vi "Process.vi"(8 "error in":errorcluster, 11 "SMO.A":refnum<class "SMO.D.lvclass">) -> (0 "error out":errorcluster, 3 "SMO.A out":refnum<class "SMO.D.lvclass">)   [LabVIEW 2013, in "SMO.D.lvclass"]
doc: "---------------------------------------------------------------\nJKI State Machine Objects™\nhttp://jki.net/state-machine-objects/\nCopyright (C) 2005-2015, JKI <info@jki.net>\nALL RIGHTS RESERVED"
uses:
  SMO.D.lvclass
  src/SMO/Typedefs/Parent Call--Enum.ctl
  src/SMO/SMO.lvclass
panel:
  # "For instructions on how to use the JKI State Machine Objects, examples and video tutorials, visit:\nhttp://jki.net/state-machine-objects/\n\nJKI State Machine Objects™\nhttp://jki.net/state-machine-objects/\nCopyright (C) 2005-2015, JKI <info@jki.net>\nALL RIGHTS RESERVED"
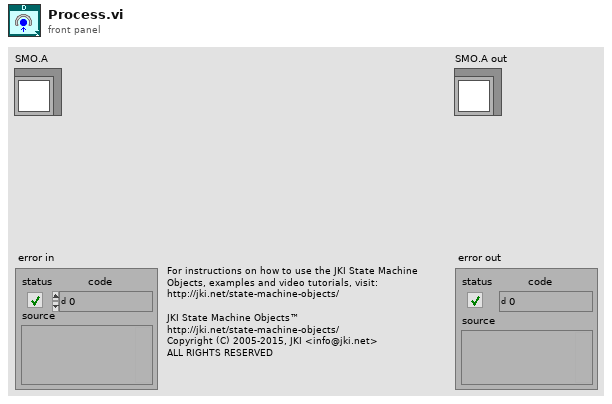
[diagram p1: front panel]
types:
  T1 = typedef "SMO.lvclass/Parent Call--Enum.ctl" = enum16{"Allows parent to run", "Does not request parent to run"}
  T2 = enum32{"invalid app kind", "Development System", "Run Time System", "Student Edition", "Embedded LabVIEW", "Evaluation", "Custom"}
  T3 = enum32{"Invalid", "Standard", "Closed", "Hidden", "Minimized", "Maximized"}
  T4 = cluster{"Core":cluster{"Current VI Reference":refnum<vi>, "Close Panel on Exit?":bool, "error":errorcluster}, "Self Ref":refnum<class "SMO.D.lvclass">, "Your string data":string, "Pump State":bool, "Valve 1 State":bool, "Flow 1 Actual":dbl, "Flow 2 Actual":dbl, "Flow 1 Target":dbl, "Flow 2 Target":dbl}
  T5 = cluster{"Current VI Reference":refnum<vi>, "Close Panel on Exit?":bool, "error":errorcluster}
  T6 = typedef "SMO.lvclass/Protected Events.ctl" = cluster{"StopProcesses":refnum<user-event>, "AbortProcesses":refnum<user-event>, "Config Changed":refnum<user-event>, "Dependency":refnum<user-event>}
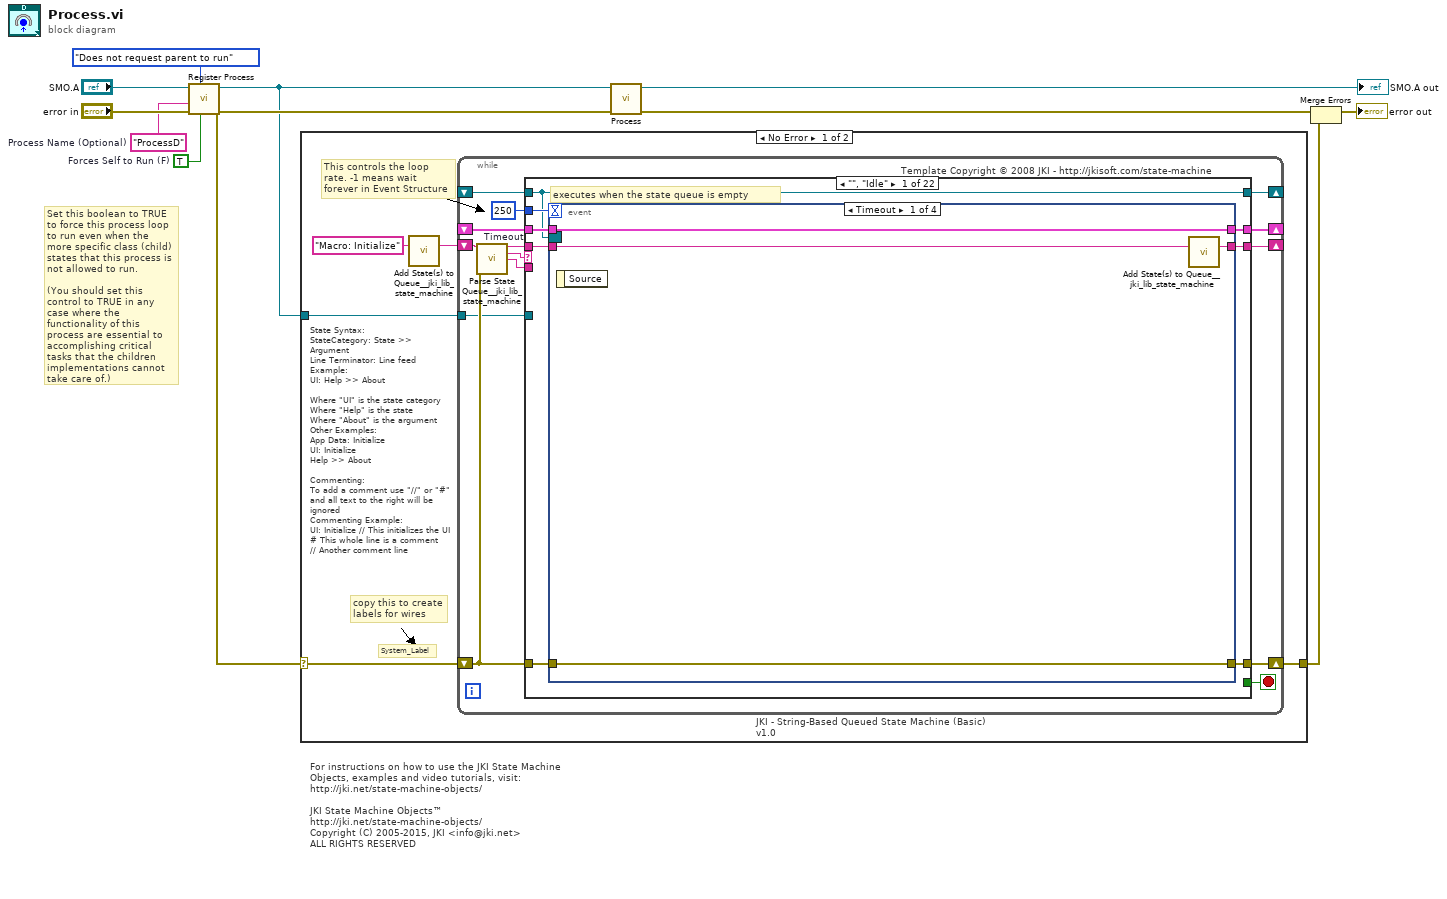
[diagram p0: block diagram]
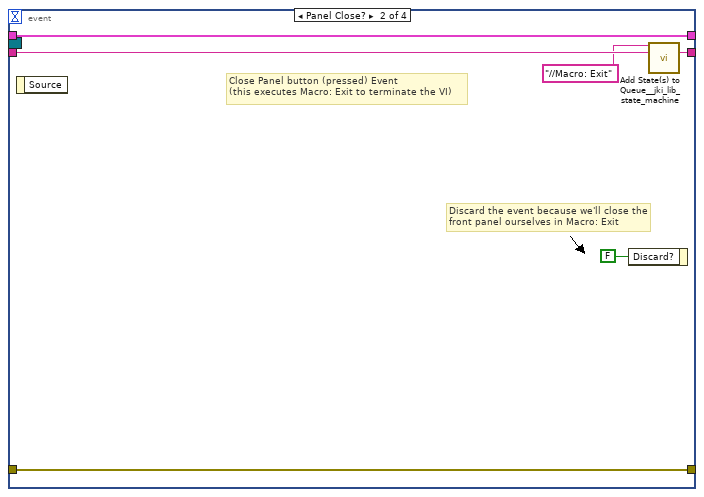
[diagram p2: hidden frame]
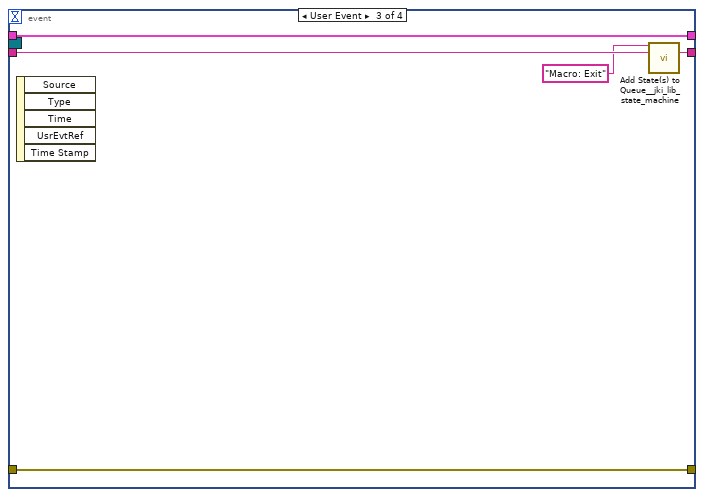
[diagram p3: hidden frame]
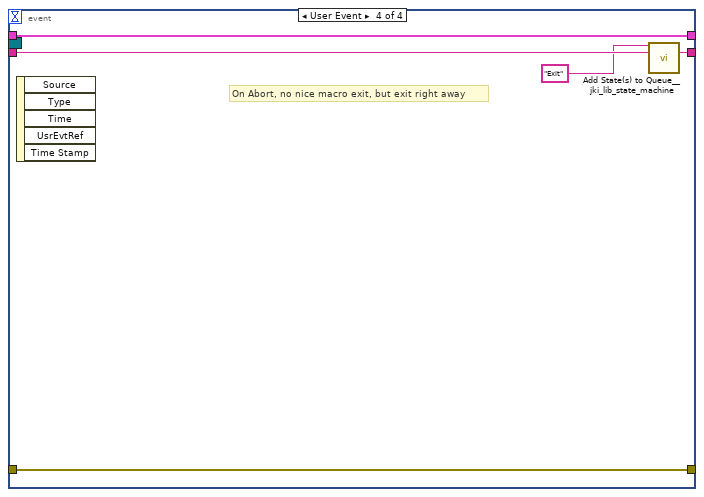
[diagram p4: hidden frame]
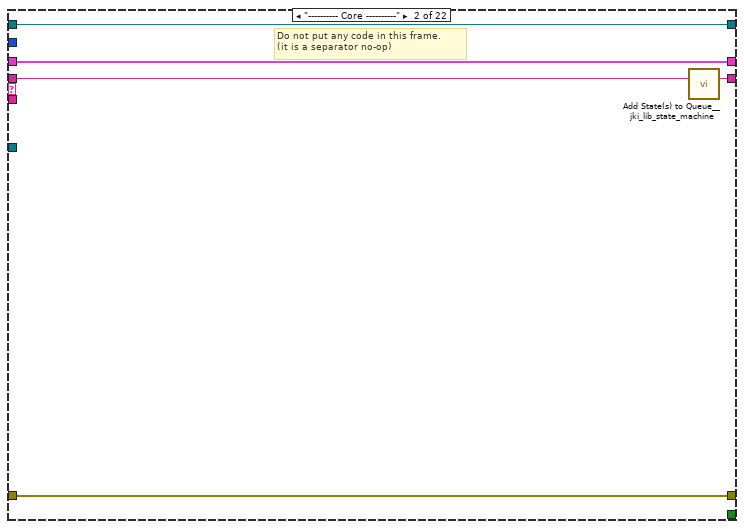
[diagram p5: hidden frame]
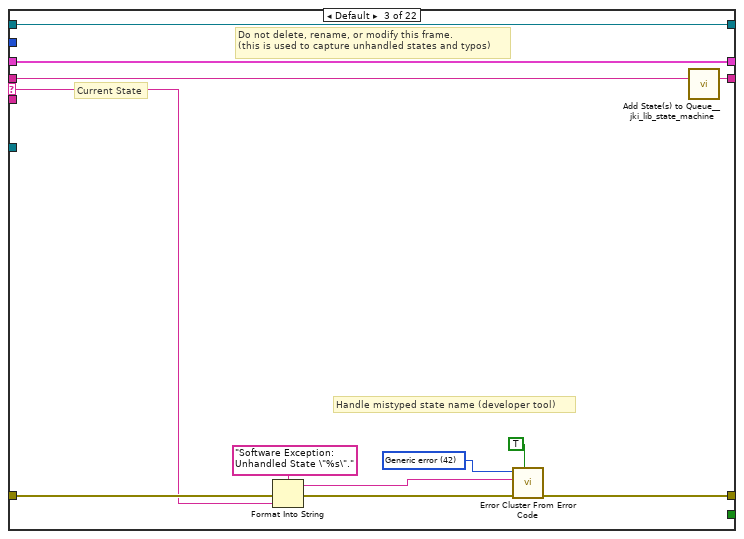
[diagram p6: hidden frame]
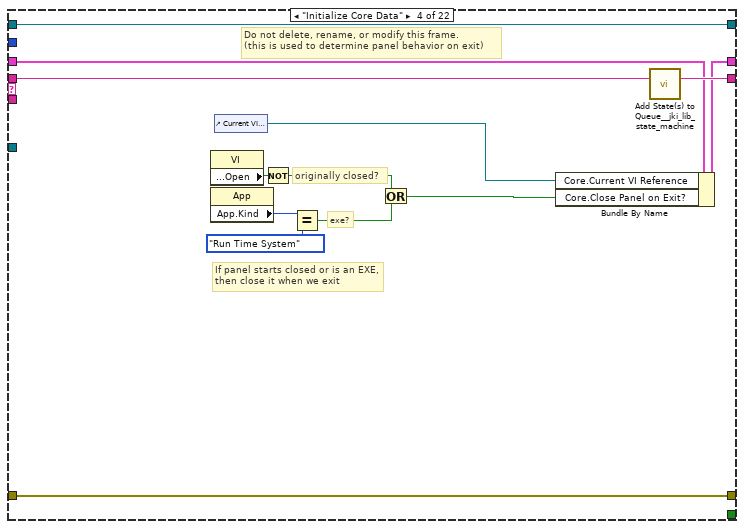
[diagram p7: hidden frame]
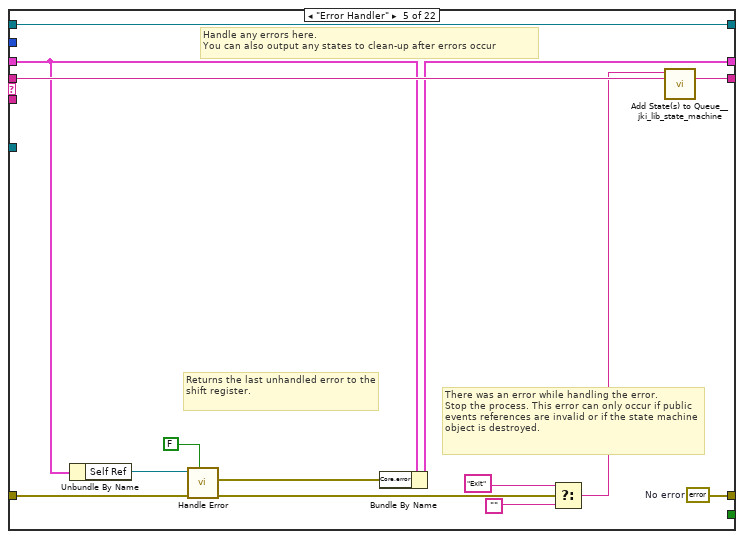
[diagram p8: hidden frame]
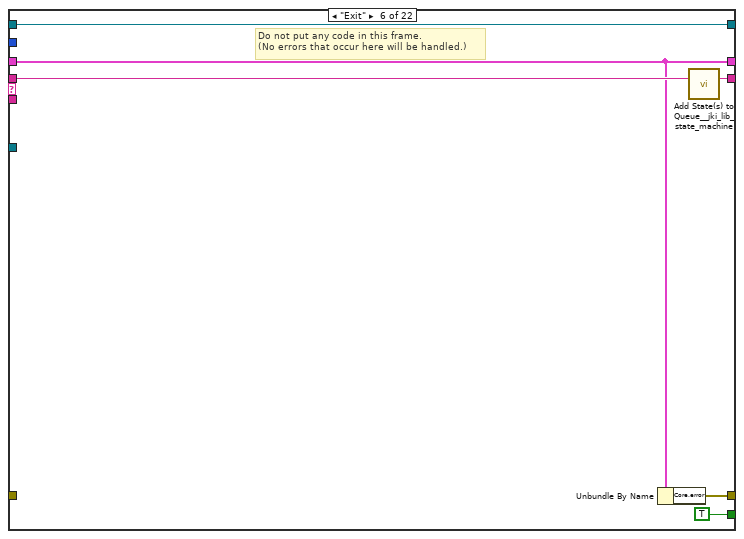
[diagram p9: hidden frame]
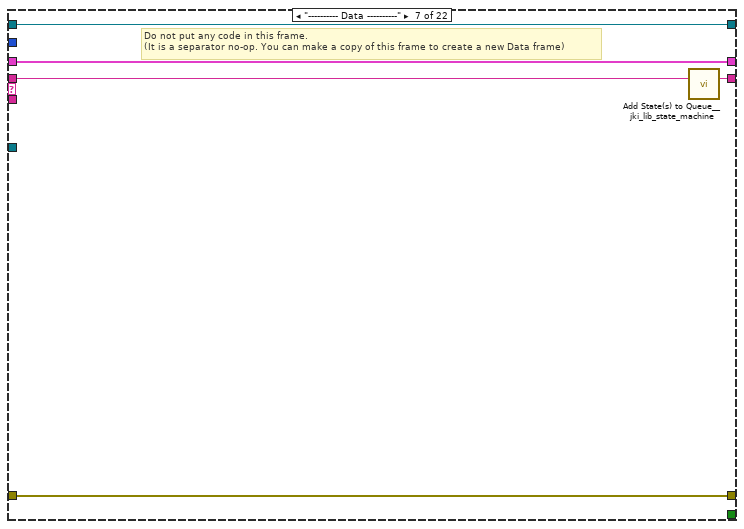
[diagram p10: hidden frame]
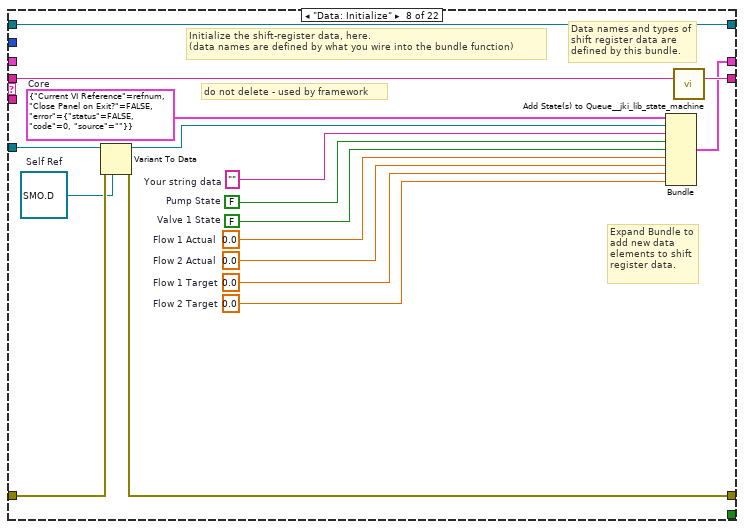
[diagram p11: hidden frame]
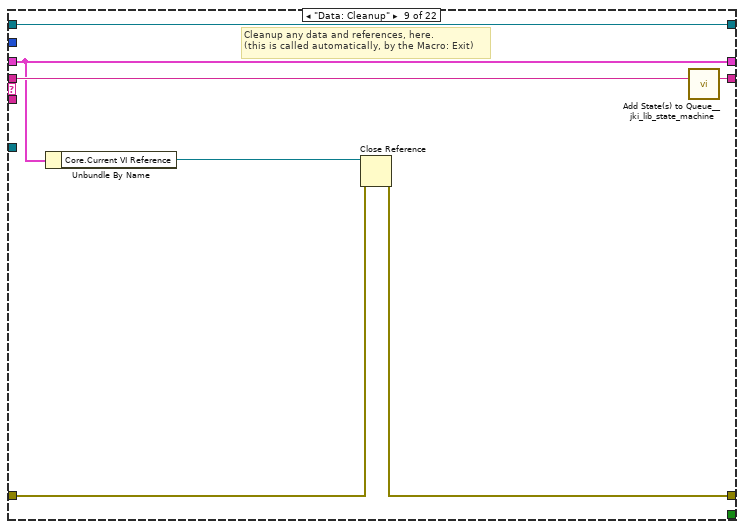
[diagram p12: hidden frame]
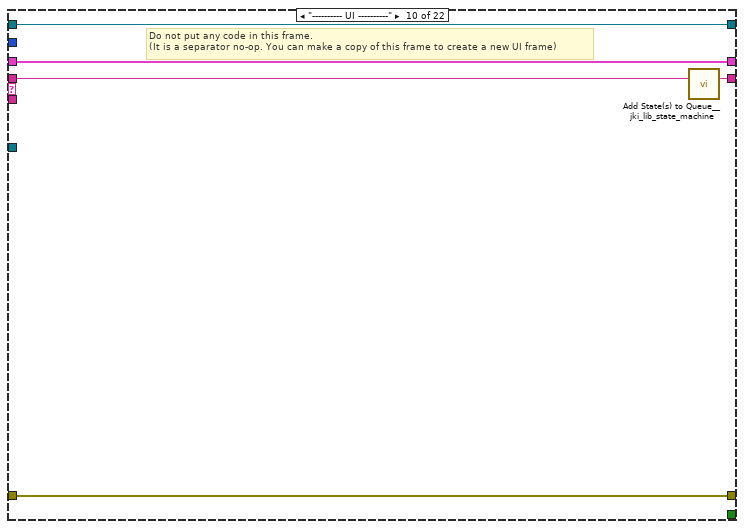
[diagram p13: hidden frame]
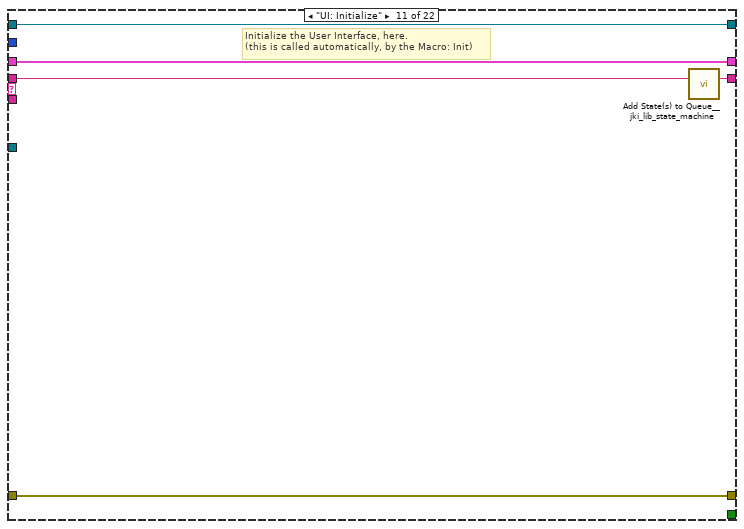
[diagram p14: hidden frame]
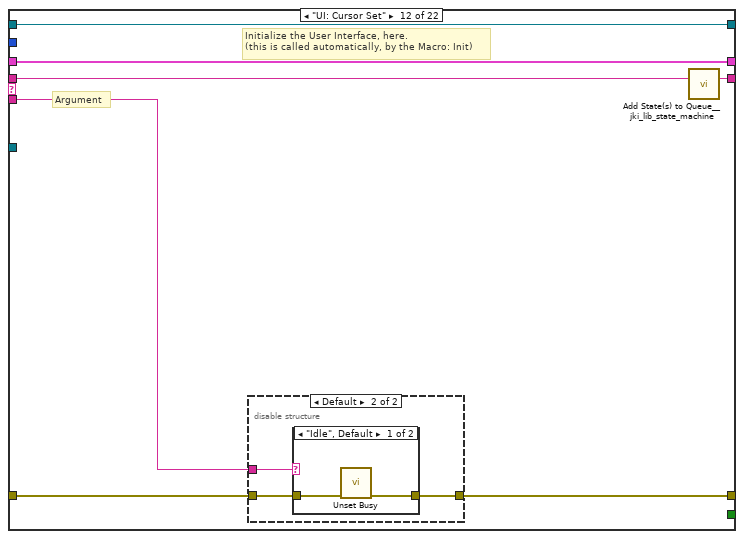
[diagram p15: hidden frame]
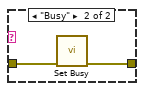
[diagram p17: hidden frame]
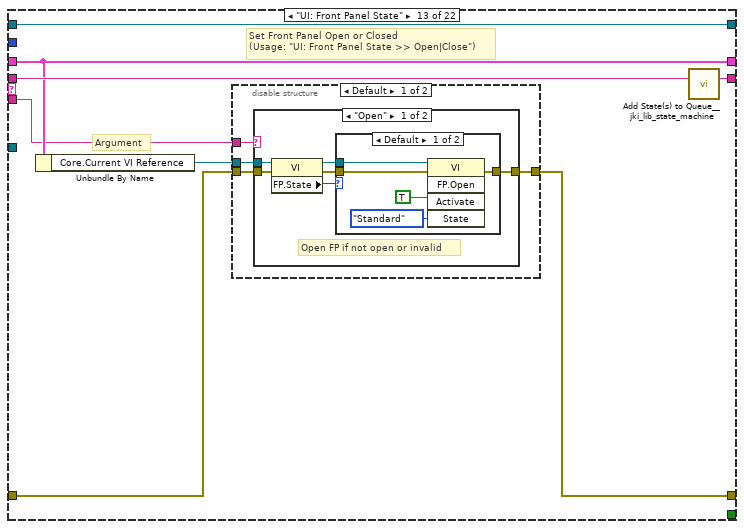
[diagram p18: hidden frame]
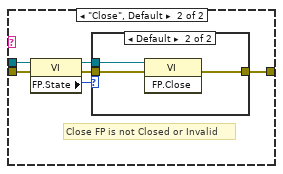
[diagram p20: hidden frame]
diagram:
  w1 = TRUE  # Forces Self to Run (F)
  w2 = "ProcessD"  # Process Name (Optional)
  # "Set this boolean to TRUE to force this process loop to run even when the more specific class (child) states that this process is not allowed to run.\n\n(You should set this control to TRUE in any case where the functionality of this process are essential to accomplishing critical tasks that the children implementations cannot take care of.)"
  # "For instructions on how to use the JKI State Machine Objects, examples and video tutorials, visit:\nhttp://jki.net/state-machine-objects/\n\nJKI State Machine Objects™\nhttp://jki.net/state-machine-objects/\nCopyright (C) 2005-2015, JKI <info@jki.net>\nALL RIGHTS RESERVED"
  n1 = call "Register Process.vi"("Forces Self to Run (F)"=w1, "Parent Call"=Parent_Call--Enum."Does not request parent to run", "error in (no error)"="error in", "Process Name (optional)"=w2, "SMO"="SMO.A") -> ("error out"=w8:errorcluster, "SMO out"=w7:refnum<class "SMO.D.lvclass">)  [unwired: 5 in]
  n2 = case shown="No Error" w8 {
    selector: w8 -> [w13 w268]
    tunnel: w7 -> [w14 _]
    tunnel: [w12 w268] -> w4
    frame No Error {
      # "State Syntax:\nStateCategory: State >> Argument\nLine Terminator: Line feed\nExample:\nUI: Help >> About\n\nWhere \"UI\" is the state category\nWhere \"Help\" is the state\nWhere \"About\" is the argument\nOther Examples:\nApp Data: Initialize\nUI: Initialize\nHelp >> About\n\nCommenting:\nTo add a comment use \"//\" or \"#\" and all text to the right will be ignored\nCommenting Example:\nUI: Initialize // This initializes the UI\n# This whole line is a comment\n// Another comment line"
      # "copy this to create labels for wires"
      # "This controls the loop rate. -1 means wait forever in Event Structure"
      # "System_Label"
      n3 = call <vilib>:"Add State(s) to Queue__jki_lib_state_machine.vi"("State(s) in (\"\")"="Macro: Initialize") -> ("States Out"=w16:string)  [unwired: 14 in]
      n4 = while "JKI - String-Based Queued State Machine (Basic) v1.0" {
        shift-right: [w23] -> _
        shift-left: _ -> [w22]
        shift-right: [w26] -> w12
        shift-left: w13 -> [w20]
        shift-right: [w25] -> _
        shift-left: w16 -> [w27]
        tunnel: w14 -> [w19]
        shift-right: [w18] -> _
        shift-left: _ -> [w17]
        stop <- w24 stop-if-true
        w21 = 250  # Timeout
        # "Template Copyright © 2008 JKI - http://jkisoft.com/state-machine"
        n5 = call <vilib>:"Parse State Queue__jki_lib_state_machine.vi"("State Queue"=w27, "Error In (no error)"=w20) -> ("Remaining States"=w29:string, "Current State"=w30:string, "Arguments"=w28:string)  [unwired: 11 in]
        n6 = case shown="\"\", \"Idle\"" w30 {
          selector: w30 -> [_ _ w65 _ _ _ _ _ _ _ _ _ _ _ _ _ _ _ _ _ _ _]
          tunnel: w29 -> [w38 w63 w69 w88 w102 w108 w113 w130 w137 w142 w147 w154 w170 w202 w211 w225 w230 w241 w246 w256 w262 w267]
          tunnel: w28 -> [_ _ _ _ _ _ _ _ _ _ _ w148 w163 _ _ _ _ _ _ _ _ _]
          tunnel: w22 -> [w36 w60 w67 w79 w93 w104 w110 _ w132 w139 w145 w152 w168 w199 w207 w216 w227 w238 w243 w254 w260 w265]
          tunnel: [w35 w61 w71 w85 w90 w103 w111 w125 w133 w140 w144 w149 w164 w200 w209 w223 w228 w232 w244 w247 w258 w263] -> w26
          tunnel: w20 -> [w34 w61 w70 w85 w94 _ w111 w126 w134 w140 w144 w150 w165 w200 w209 w223 w228 w233 w244 w248 w258 w263]
          tunnel: [w37 w62 w68 w87 w101 w107 w112 w129 w136 w141 w146 w153 w169 w201 w210 w224 w229 w240 w245 w255 w261 w266] -> w25
          tunnel: [_ _ _ _ _ TRUE _ _ _ _ _ _ _ _ _ _ _ _ _ _ _ _] -> w24
          tunnel: [w33 w60 w67 w86 w92 w104 w110 w128 w132 w139 w145 w152 w168 w199 w207 w216 w227 w238 w243 w254 w260 w265] -> w23
          tunnel: w21 -> [w32 _ _ _ _ _ _ _ _ _ _ _ _ _ _ _ _ _ _ _ _ _]
          tunnel: w19 -> [_ _ _ _ _ _ _ w123 _ _ _ _ _ _ _ _ _ _ _ _ _ _]
          tunnel: [w31 w59 w64 w76 w100 w105 w109 w121 w131 w138 w143 w151 w167 w198 w208 w217 w226 w239 w242 w251 w259 w264] -> w18
          tunnel: w17 -> [w31 w59 w64 w76 w100 w105 w109 w121 w131 w138 w143 w151 w167 w198 w208 w217 w226 w239 w242 _ w259 w264]
          frame "", "Idle" {
            # "executes when the state queue is empty"
            n7 = event shown="[0] Timeout" {
              selector: w31 -> [_ _ _ _]
              dyn-events: _ -> [_ _ _ _]
              timeout: w32 -> [_ _ _ _]
              tunnel: w38 -> [w42 w48 w53 w58]
              tunnel: [w41 w47 w52 w57] -> w37
              tunnel: w36 -> [w39 w45 w50 w55]
              tunnel: [w40 w46 w51 w56] -> w35
              tunnel: w34 -> [w40 w46 w51 w56]
              tunnel: [w39 w45 w50 w55] -> w33
              event Timeout {
                n8 = event-data() -> ()  [unwired: 1 in, 1 out]
                n9 = call <vilib>:"Add State(s) to Queue__jki_lib_state_machine.vi"("State(s) in (\"\")"=w42) -> ("States Out"=w41:string)  [unwired: 14 in]
              }
              event Panel Close? {
                # "Discard the event because we'll close the front panel ourselves in Macro: Exit"
                # "Close Panel button (pressed) Event\n(this executes Macro: Exit to terminate the VI)"
                n10 = event-data() -> ()  [unwired: 1 in, 1 out]
                n11 = event-data("Discard?"=FALSE) -> ()  [unwired: 1 in, 1 out]
                n12 = call <vilib>:"Add State(s) to Queue__jki_lib_state_machine.vi"("State(s) in Front (\"\")"="//Macro: Exit", "State(s) in (\"\")"=w48) -> ("States Out"=w47:string)  [unwired: 13 in]
              }
              event User Event {
                n13 = event-data() -> ()  [unwired: 1 in, 5 out]
                n14 = call <vilib>:"Add State(s) to Queue__jki_lib_state_machine.vi"("State(s) in Front (\"\")"="Macro: Exit", "State(s) in (\"\")"=w53) -> ("States Out"=w52:string)  [unwired: 13 in]
              }
              event User Event {
                # "On Abort, no nice macro exit, but exit right away"
                n15 = event-data() -> ()  [unwired: 1 in, 5 out]
                n16 = call <vilib>:"Add State(s) to Queue__jki_lib_state_machine.vi"("State(s) in Front (\"\")"="Exit", "State(s) in (\"\")"=w58) -> ("States Out"=w57:string)  [unwired: 13 in]
              }
            }
          }
          frame "---------- Core ----------" {
            # "Do not put any code in this frame.\n(it is a separator no-op)"
            n17 = call <vilib>:"Add State(s) to Queue__jki_lib_state_machine.vi"("State(s) in (\"\")"=w63) -> ("States Out"=w62:string)  [unwired: 14 in]
          }
          frame Default {
            w74 = 42 items=["No error", "Argument error", "Memory is full", "Out of zone", "End of file", "File already open", "Generic file I/O error", "File not found", "File permission error", "Disk is full", "Duplicate path", "Too many files open", "System feature not enabled", "Resource file not found", "Cannot add resource", "Resource not found", "Image not found", "Image memory error", "Pen does not exist", "Config type invalid", "Config token not found", "Config parse error", "Config memory error", "Bad external code format", "Bad external code offset", "External code not present", "Null window", "Destroy window error", "Null menu", "Print aborted", "Bad print record", "Print driver error", "Windows error during printing", "Memory error during printing", "Print dialog error", "Generic print error", "Invalid device refnum", "Device not found", "Device parameter error", "Device unit error", "Cannot open device", "Device call aborted", "Generic error", "Cancelled by user", "Object ID too low", "Object ID too high", "Object not in heap", "Unknown heap", "Unknown object (invalid DefProc)", "Unknown object (DefProc not in table)", "Message out of range", "Invalid (null) method", "Unknown message", "Manager call not supported", "Bad address", "Network operation in progress", "Network operation timed out", "Connection is busy", "Network attribute not supported", "Network error", "Address in use", "System out of memory", "Connection aborted", "Connection refused", "Not connected", "Already connected", "Connection closed", "Initialization error (interapplication manager)", "Bad occurrence", "Wait on unbound occurrence handler", "Occurrence queue overflow", "Datalog type conflict", "Unused", "Unrecognized type (interapplication manager)", "Memory corrupt", "Failed to make temporary DLL", "Old CIN version", "Drag socket not found", "Failed to load drop-object", "Failed to register OLE object", "Failed to release OLE object", "Format specifier type mismatch", "Unknown format specifier", "Too few format specifiers", "Too many format specifiers", "Scan failed", "Newer CIN version", "Error converting to variant", "Runtime menu error", "Password tampered", "Variant attribute not found", "Incompatible variant data type", "Event data is not available", "Event Store is not present", "Occurrence is not found", "Event Queue is not created", "Event info is not available", "Refnum passed is NULL", "Error retrieving Class GUID", "Error retrieving CoClass GUID", "Error retrieving TypeLib GUID.", "Bad built application magic bytes.", "Specific driver is different from the specific driver associated with the Logical Name.", "There is no session opened to the class driver.", "Max Error", "MAX - Error with config objects", "MAX - Error loading configuration", "MAX - Group not supported"]
            # "Current State"
            # "Do not delete, rename, or modify this frame.\n(this is used to capture unhandled states and typos)"
            # "Handle mistyped state name (developer tool)"
            n18 = Format Into String(format string="Software Exception: Unhandled State \"%s\"." ("message"), error in=w70, w65) -> (resulting string=w73:string, error out=w72:errorcluster)  [unwired: 1 in]
            n19 = call <vilib>:"Error Cluster From Error Code.vi"("show call chain? (False)"=TRUE, "error in (no error)"=w72, "error message (\"\")"=w73, "error code (0)"=w74) -> ("error out"=w71:errorcluster)  [unwired: 5 in]
            n20 = call <vilib>:"Add State(s) to Queue__jki_lib_state_machine.vi"("State(s) in (\"\")"=w69) -> ("States Out"=w68:string)  [unwired: 14 in]
          }
          frame "Initialize Core Data" {
            # "Do not delete, rename, or modify this frame.\n(this is used to determine panel behavior on exit)"
            # "originally closed?"
            # "exe?"
            # "If panel starts closed or is an EXE, then close it when we exit"
            n21 = property class="VI"() -> ("Front Panel.Open"=w84:bool)  [unwired: 2 in, 2 out]
            n22 = property class="App"() -> ("App.Kind"=w83:T2)  [unwired: 2 in, 2 out]
            n23 = control-ref of="Current VI Reference"() -> (w77:refnum<vi>)
            n24 = Not(x=w84) -> (.not. x?=w81:bool)
            n25 = Equal?(x=w83, y=T2."Run Time System" ("Application:Kind")) -> (x = y?=w80:bool)
            n26 = Or(x=w81, y=w80) -> (x .or. y?=w78:bool)
            n27 = Bundle By Name(cluster=w79, "Core.Current VI Reference"=w77, "Core.Close Panel on Exit?"=w78) -> (w86:T4)
            n28 = call <vilib>:"Add State(s) to Queue__jki_lib_state_machine.vi"("State(s) in (\"\")"=w88) -> ("States Out"=w87:string)  [unwired: 14 in]
          }
          frame "Error Handler" {
            w90 = errorcluster {"status"=FALSE, "code"=0, "source"=""}  # No error
            # "Returns the last unhandled error to the shift register."
            # "There was an error while handling the error.\nStop the process. This error can only occur if public events references are invalid or if the state machine object is destroyed."
            # "Handle any errors here.\nYou can also output any states to clean-up after errors occur"
            n29 = Unbundle By Name(w93) -> ("Self Ref"=w95:refnum<class "SMO.D.lvclass">)
            n30 = call-dynamic "Handle Error.vi"("Stop on Unhandled Error (T)"=FALSE, "error in"=w94, "SMO"=w95) -> ("handling error"=w97:errorcluster, "Unhandled error"=w96:errorcluster)  [unwired: 6 in, 1 out]
            n31 = Bundle By Name(cluster=w93, "Core.error"=w96) -> (w92:T4)
            n32 = Select(t="Exit", s=w97, f="") -> (s? t:f=w91:string)
            n33 = call <vilib>:"Add State(s) to Queue__jki_lib_state_machine.vi"("State(s) in Front (\"\")"=w91, "State(s) in (\"\")"=w102) -> ("States Out"=w101:string)  [unwired: 13 in]
          }
          frame "Exit" {
            # "Do not put any code in this frame.\n(No errors that occur here will be handled.)"
            n34 = Unbundle By Name(w104) -> ("Core.error"=w103:errorcluster)
            n35 = call <vilib>:"Add State(s) to Queue__jki_lib_state_machine.vi"("State(s) in (\"\")"=w108) -> ("States Out"=w107:string)  [unwired: 14 in]
          }
          frame "---------- Data ----------" {
            # "Do not put any code in this frame.\n(It is a separator no-op. You can make a copy of this frame to create a new Data frame)"
            n36 = call <vilib>:"Add State(s) to Queue__jki_lib_state_machine.vi"("State(s) in (\"\")"=w113) -> ("States Out"=w112:string)  [unwired: 14 in]
          }
          frame "Data: Initialize" {
            w114 = T5 {"Current VI Reference"=refnum, "Close Panel on Exit?"=FALSE, "error"={"status"=FALSE, "code"=0, "source"=""}}  # Core
            w115 = 0.0  # Flow 2 Target
            w116 = 0.0  # Flow 1 Target
            w117 = 0.0  # Flow 2 Actual
            w118 = 0.0  # Flow 1 Actual
            w119 = FALSE  # Valve 1 State
            w120 = FALSE  # Pump State
            w124 = refnum<class "SMO.D.lvclass"> refnum  # Self Ref
            w127 = ""  # Your string data
            # "do not delete - used by framework"
            # "Expand Bundle to add new data elements to shift register data."
            # "Data names and types of shift register data are defined by this bundle."
            # "Initialize the shift-register data, here.\n(data names are defined by what you wire into the bundle function)"
            n37 = Variant To Data(error in=w126, type=w124, Variant=w123) -> (data=w122:refnum<class "SMO.D.lvclass">, error out=w125:errorcluster)
            n38 = Bundle("Core"=w114, "Self Ref"=w122, "Your string data"=w127, "Pump State"=w120, "Valve 1 State"=w119, "Flow 1 Actual"=w118, "Flow 2 Actual"=w117, "Flow 1 Target"=w116, "Flow 2 Target"=w115) -> (w128:T4)  [unwired: 1 in]
            n39 = call <vilib>:"Add State(s) to Queue__jki_lib_state_machine.vi"("State(s) in (\"\")"=w130) -> ("States Out"=w129:string)  [unwired: 14 in]
          }
          frame "Data: Cleanup" {
            # "Cleanup any data and references, here.\n(this is called automatically, by the Macro: Exit)"
            n40 = Unbundle By Name(w132) -> ("Core.Current VI Reference"=w135:refnum<vi>)
            n41 = Close Reference(reference=w135, error in (no error)=w134) -> (error out=w133:errorcluster)
            n42 = call <vilib>:"Add State(s) to Queue__jki_lib_state_machine.vi"("State(s) in (\"\")"=w137) -> ("States Out"=w136:string)  [unwired: 14 in]
          }
          frame "---------- UI ----------" {
            # "Do not put any code in this frame.\n(It is a separator no-op. You can make a copy of this frame to create a new UI frame)"
            n43 = call <vilib>:"Add State(s) to Queue__jki_lib_state_machine.vi"("State(s) in (\"\")"=w142) -> ("States Out"=w141:string)  [unwired: 14 in]
          }
          frame "UI: Initialize" {
            # "Initialize the User Interface, here.\n(this is called automatically, by the Macro: Init)"
            n44 = call <vilib>:"Add State(s) to Queue__jki_lib_state_machine.vi"("State(s) in (\"\")"=w147) -> ("States Out"=w146:string)  [unwired: 14 in]
          }
          frame "UI: Cursor Set" {
            # "Argument"
            # "Initialize the User Interface, here.\n(this is called automatically, by the Macro: Init)"
            n45 = disable-structure shown="Default" {
              disable-tunnel: w150 -> [w155 w158]
              disable-tunnel: [w155 w157] -> w149
              disable-tunnel: w148 -> [_ w156]
              frame condition #0 {
              }
              frame condition #1 (active) {
                n46 = case shown="\"Idle\", Default" w156 {
                  tunnel: w158 -> [w160 w162]
                  tunnel: [w159 w161] -> w157
                  frame "Idle", Default {
                    n47 = call <vilib>:"Unset Busy.vi"("error in (no error)"=w160) -> ("error out"=w159:errorcluster)  [unwired: 10 in]
                  }
                  frame "Busy" {
                    n48 = call <vilib>:"Set Busy.vi"("error in (no error)"=w162) -> ("error out"=w161:errorcluster)  [unwired: 9 in, 1 out]
                  }
                }
              }
            }
            n49 = call <vilib>:"Add State(s) to Queue__jki_lib_state_machine.vi"("State(s) in (\"\")"=w154) -> ("States Out"=w153:string)  [unwired: 14 in]
          }
          frame "UI: Front Panel State" {
            # "Argument"
            # "Set Front Panel Open or Closed\n(Usage: \"UI: Front Panel State >> Open|Close\")"
            n50 = Unbundle By Name(w168) -> ("Core.Current VI Reference"=w166:refnum<vi>)
            n51 = disable-structure shown="Default" {
              disable-tunnel: w165 -> [w174 w197]
              disable-tunnel: [w173 w197] -> w164
              disable-tunnel: w166 -> [w172 _]
              disable-tunnel: w163 -> [w171 _]
              frame condition #0 (active) {
                n52 = case shown="\"Open\"" w171 {
                  tunnel: w174 -> [w178 w191]
                  tunnel: [w180 w192] -> w173
                  tunnel: w172 -> [w179 w189]
                  frame "Open" {
                    # "Open FP if not open or invalid"
                    n53 = property class="VI"(reference=w179, error in=w178) -> (reference out=w176:refnum<vi>, error out=w177:errorcluster, "FP.State"=w175:T3)
                    n54 = case shown="Default" w175 {
                      tunnel: [w183 w186] -> w180
                      tunnel: w177 -> [w182 w186]
                      tunnel: w176 -> [w181 _]
                      frame Default {
                        n55 = invoke class="VI" method="FP.Open"(reference=w181, error in=w182, "Activate"=TRUE, "State"=T3."Standard") -> (error out=w183:errorcluster)  [unwired: 1 in, 4 out]
                      }
                      frame "Invalid", "Standard" {
                      }
                    }
                  }
                  frame "Close", Default {
                    # "Close FP is not Closed or Invalid"
                    n56 = property class="VI"(reference=w189, error in=w191) -> (reference out=w188:refnum<vi>, error out=w190:errorcluster, "FP.State"=w187:T3)
                    n57 = case shown="Default" w187 {
                      tunnel: [w193 w196] -> w192
                      tunnel: w190 -> [w193 w195]
                      tunnel: w188 -> [_ w194]
                      frame "Invalid", "Closed" {
                      }
                      frame Default {
                        n58 = invoke class="VI" method="FP.Close"(reference=w194, error in=w195) -> (error out=w196:errorcluster)  [unwired: 1 in, 2 out]
                      }
                    }
                  }
                }
              }
              frame condition #1 {
              }
            }
            n59 = call <vilib>:"Add State(s) to Queue__jki_lib_state_machine.vi"("State(s) in (\"\")"=w170) -> ("States Out"=w169:string)  [unwired: 14 in]
          }
          frame "---------- Macro ----------" {
            # "Do not put any code in this frame.\n(It is a separator no-op. You can make a copy of this frame to create a new Macro frame)"
            n60 = call <vilib>:"Add State(s) to Queue__jki_lib_state_machine.vi"("State(s) in (\"\")"=w202) -> ("States Out"=w201:string)  [unwired: 14 in]
          }
          frame "Macro: Initialize" {
            w205 = "UI: Initialize\n//UI: Front Panel State >> Open"  # UI: Initialize //UI: Front Panel State >> Open
            # "Initialization Macro\n(This is called once, when the VI starts)"
            n61 = call <vilib>:"Add State(s) to Queue__jki_lib_state_machine.vi"("State(s) in Front (\"\")"="Data: Initialize\nInitialize Core Data\nEvents: Register", "State(s) in (\"\")"="Process: Sync", "State(s) at Back (\"\")"=w205) -> ("States Out"=w204:string)  [unwired: 12 in]
            n62 = call <vilib>:"Add State(s) to Queue__jki_lib_state_machine.vi"("State(s) in Front (\"\")"=w204, "State(s) in (\"\")"=w211) -> ("States Out"=w210:string)  [unwired: 13 in]
          }
          frame "Macro: Exit" {
            # "Exit Macro\n(This is called once, when the VI exits)"
            n63 = Unbundle By Name(w216) -> ("Core.Close Panel on Exit?"=w222:bool)
            n64 = Select(t="//UI: Front Panel State >> Close", s=w222, f="") -> (s? t:f=w219:string)
            n65 = call <vilib>:"Add State(s) to Queue__jki_lib_state_machine.vi"("State(s) in Front (\"\")"="Data: Cleanup\nEvents: Unregister", "State(s) in (\"\")"="Process: Sync", "State(s) at Back (\"\")"="Exit") -> ("States Out"=w213:string)  [unwired: 12 in]
            n66 = call <vilib>:"Add State(s) to Queue__jki_lib_state_machine.vi"("State(s) in (\"\")"=w219, "State(s) at Back (\"\")"=w213) -> ("States Out"=w218:string)  [unwired: 13 in]
            n67 = call <vilib>:"Add State(s) to Queue__jki_lib_state_machine.vi"("State(s) in Front (\"\")"=w218, "State(s) in (\"\")"=w225) -> ("States Out"=w224:string)  [unwired: 13 in]
          }
          frame "---------- Process ----------" {
            # "Template Separator\n(You can make a copy of, or modify, this frame)"
            n68 = call <vilib>:"Add State(s) to Queue__jki_lib_state_machine.vi"("State(s) in (\"\")"=w230) -> ("States Out"=w229:string)  [unwired: 14 in]
          }
          frame "Process: Sync" {
            # "Template Separator\n(You can make a copy of, or modify, this frame)"
            n69 = Unbundle By Name(w238) -> ("Self Ref"=w234:refnum<class "SMO.D.lvclass">)
            n70 = call "WaitOnProcessSync.vi"("error in (no error)"=w233, "SMO"=w234) -> ("error out"=w232:errorcluster, "Don't run?"=w237:bool)  [unwired: 7 in, 1 out]
            n71 = Select(t="Data: Cleanup\nEvents: Unregister\nExit", s=w237, f="") -> (s? t:f=w231:string)
            n72 = call <vilib>:"Add State(s) to Queue__jki_lib_state_machine.vi"("State(s) in Front (\"\")"=w231, "State(s) in (\"\")"=w241) -> ("States Out"=w240:string)  [unwired: 13 in]
          }
          frame "---------- Events ----------" {
            # "Template Separator\n(You can make a copy of, or modify, this frame)"
            n73 = call <vilib>:"Add State(s) to Queue__jki_lib_state_machine.vi"("State(s) in (\"\")"=w246) -> ("States Out"=w245:string)  [unwired: 14 in]
          }
          frame "Events: Register" {
            # "Self Public Events"
            # "Base Class Protected Events"
            # "Your code here.\n(You can make a copy of, or modify, this frame)"
            n74 = Unbundle By Name(w254) -> ("Self Ref"=w253:refnum<class "SMO.D.lvclass">)
            n75 = call "GetProtectedEvents.vi"("SMO"=w253) -> ("error out"=w249:errorcluster, "SMO Protected Events"=w252:T6)  [unwired: 8 in, 1 out]
            n76 = register-events(w252) -> (reference out=w251:refnum<event-registration>, error out=w250:errorcluster)  [unwired: 2 in]
            n77 = Merge Errors(w248, w250, w249) -> (w247:errorcluster)
            n78 = call <vilib>:"Add State(s) to Queue__jki_lib_state_machine.vi"("State(s) in (\"\")"=w256) -> ("States Out"=w255:string)  [unwired: 14 in]
          }
          frame "Events: Unregister" {
            # "Your code here.\n(You can make a copy of, or modify, this frame)"
            n79 = Unregister For Events(event registration refnum=w259, error in=w258) -> (error out=w257:errorcluster)
            n80 = call <vilib>:"Clear Errors.vi"("error in (no error)"=w257) -> ()  [unwired: 6 in, 1 out]
            n81 = call <vilib>:"Add State(s) to Queue__jki_lib_state_machine.vi"("State(s) in (\"\")"=w262) -> ("States Out"=w261:string)  [unwired: 14 in]
          }
          frame "---------- API ----------" {
            n82 = call <vilib>:"Add State(s) to Queue__jki_lib_state_machine.vi"("State(s) in (\"\")"=w267) -> ("States Out"=w266:string)  [unwired: 14 in]
          }
        }
      }
    }
    frame Error {
    }
  }
  n83 = call-parent "Process.vi"("error in"=w8, "SMO"=w7) -> ("error out"=w5:errorcluster, "SMO out"=→"SMO.A out":refnum<class "SMO.D.lvclass">)  [unwired: 8 in]
  n84 = Merge Errors(w5, w4) -> (→"error out":errorcluster)
